vi "Array Element Count.vi"(0 "Array":variant[](array[variant]), 1 "Element":variant) -> (2 "Count":i16)   [LabVIEW 2017]
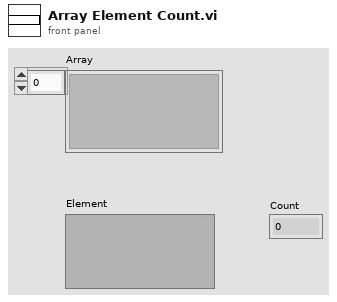
[diagram p1: front panel]
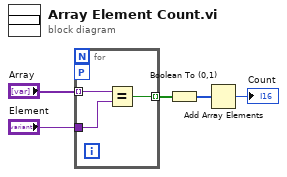
[diagram p0: block diagram]
diagram:
  n1 = for {
    tunnel: "Array" -> [w8] mode=indexing
    tunnel: "Element" -> [w7]
    tunnel: [w6] -> w3 mode=indexing
    workers-P: _ -> [_]
    n2 = Equal?(x=w8, y=w7) -> (x = y?=w6:bool)
  }
  n3 = Boolean To (0,1)(Boolean=w3) -> (0, 1=w2:i16[])
  n4 = Add Array Elements(numeric array=w2) -> (sum=→"Count":i16)
